vi "get.vi"(8 "error in (no error)":errorcluster, 10 "index":i32, 11 "CareTaker in":refnum<class "CareTaker.lvclass">) -> (0 "error out":errorcluster, 2 "Memento.lvclass":refnum<class "Memento.lvclass">, 3 "CareTaker out":refnum<class "CareTaker.lvclass">)   [LabVIEW 2018, in "CareTaker.lvclass"]
uses:
  CareTaker.lvclass
  Memento Class/Memento.lvclass
  CareTaker.lvclass/CareTaker.ctl
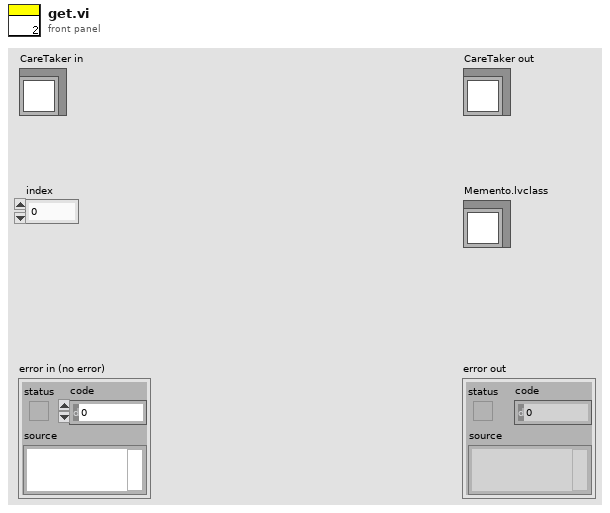
[diagram p1: front panel]
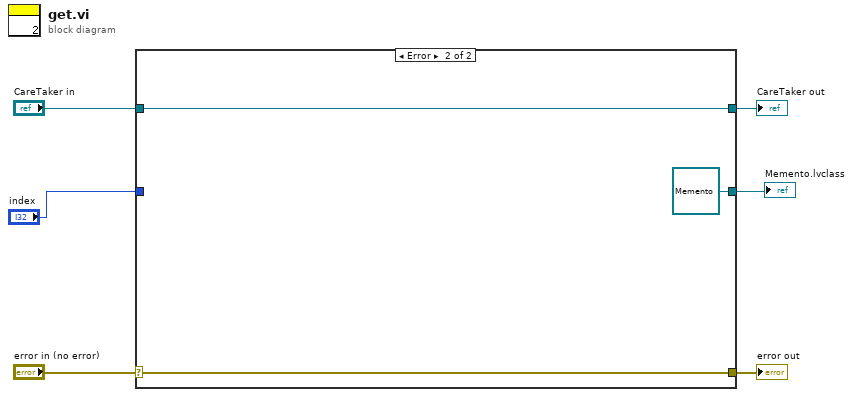
[diagram p0: block diagram]
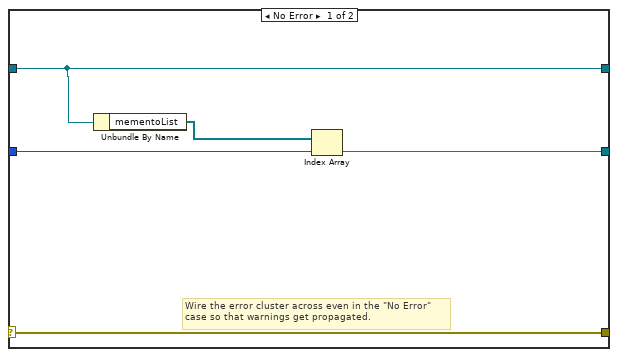
[diagram p2: hidden frame]
diagram:
  n1 = case shown="Error" "error in (no error)" {
    selector: "error in (no error)" -> [w11 w14]
    tunnel: [w11 w14] -> w5
    tunnel: [w10 w13] -> w3
    tunnel: "CareTaker in" -> [w10 w13]
    tunnel: "index" -> [w8 _]
    tunnel: [w7 refnum<class "Memento.lvclass"> refnum ("Memento.lvclass")] -> w1
    frame No Error {
      # "Wire the error cluster across even in the \"No Error\"\ncase so that warnings get propagated."
      n2 = Unbundle By Name(w10) -> ("mementoList"=w9:refnum<class "Memento.lvclass">[])
      n3 = Index Array(array=w9, index=w8) -> (element=w7:refnum<class "Memento.lvclass">)
    }
    frame Error {
    }
  }
  "error out" <- w5
  "CareTaker out" <- w3
  "Memento.lvclass" <- w1
